vi "AB_Engine_RESTful_Validate_Template_Syntax.vi"(11 "RESTful VI routing template in":T1) -> (2 "valid syntax":bool)   [LabVIEW 2020]
uses:
  <vilib>/AppBuilder/AB_Classes/RESTful/AB_RESTful_RoutingTemplate.ctl
  <vilib>/AppBuilder/AB_Classes/RESTful/AB_RESTful_RoutingType.ctl
  <vilib>/AppBuilder/AB_Classes/RESTful/AB_RESTful_HTTPMethodType.ctl
  <resource>/ws_ade.dll
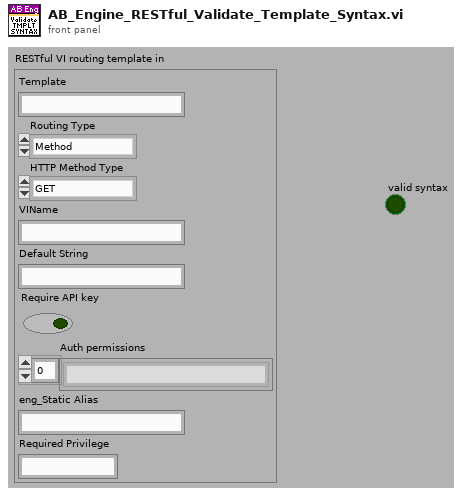
[diagram p1: front panel]
types:
  T1 = typedef "AB_RESTful_RoutingTemplate.ctl" = cluster{"Template":string, "Routing Type":T2, "HTTP Method Type":T3, "VIName":string, "Default String":string, "Require API key":bool, "Auth permissions":string[], "eng_Static Alias":string, "Required Privilege":string}
  T2 = typedef "AB_RESTful_RoutingType.ctl" = enum32{"Method", "Static"}
  T3 = typedef "AB_RESTful_HTTPMethodType.ctl" = enum32{"GET", "POST", "PUT", "DELETE"}
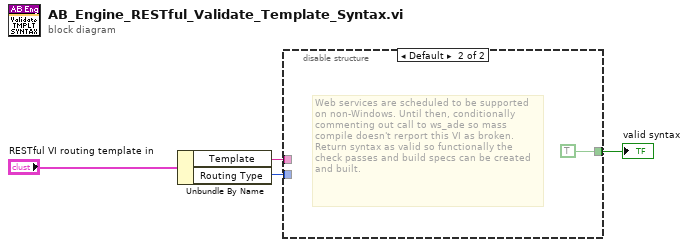
[diagram p0: block diagram]
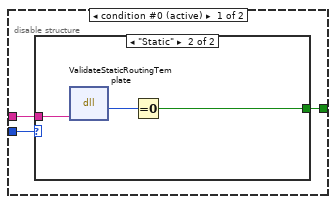
[diagram p2: hidden frame]
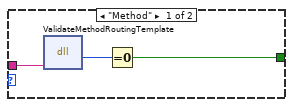
[diagram p3: hidden frame]
diagram:
  n1 = Unbundle By Name("RESTful VI routing template in") -> ("Template"=w2:string, "Routing Type"=w3:T2)
  n2 = disable-structure shown="Default" {
    disable-tunnel: w3 -> [w7 _]
    disable-tunnel: w2 -> [w6 _]
    disable-tunnel: [w5 TRUE] -> w1
    frame condition #0 (active) {
      n3 = case shown="\"Static\"" w7 {
        tunnel: w6 -> [w10 w13]
        tunnel: [w8 w11] -> w5
        frame "Method" {
          n4 = dll-call lib="e:/builds/penguin/labview/branches/2020/dev/dist/resource/ws_ade.dll" fn="ValidateMethodRoutingTemplate"("StringToParse"=w10) -> ("return type"=w9:i32)  [unwired: 4 in, 2 out]
          n5 = Equal To 0?(x=w9) -> (x = 0?=w8:bool)
        }
        frame "Static" {
          n6 = dll-call lib="e:/builds/penguin/labview/branches/2020/dev/dist/resource/ws_ade.dll" fn="ValidateStaticRoutingTemplate"("StringToParse"=w13) -> ("return type"=w12:i32)  [unwired: 4 in, 2 out]
          n7 = Equal To 0?(x=w12) -> (x = 0?=w11:bool)
        }
      }
    }
    frame condition #1 {
      # "Web services are scheduled to be supported on non-Windows. Until then, conditionally commenting out call to ws_ade so mass compile doesn't rerport this VI as broken. Return syntax as valid so functionally the check passes and build specs can be created and built."
    }
  }
  "valid syntax" <- w1
